vi "Fetch Data (SubVI).vi"(4 "error IN":errorcluster, 7 "query string":string="SELECT * FROM dbo.ThreatCalibers") -> (0 "error OUT":errorcluster, 3 "recordset data":string[][](array[string]))   [LabVIEW 2015]
uses:
  <vilib>/addons/database/Connection.llb/DB Tools Open Connec (Path).vi
  <vilib>/addons/database/Connection.llb/Conn Execute.vi
  <vilib>/addons/database/Recordset.llb/Rec Destroy - Connection.vi
  <vilib>/addons/database/NI_Database_API.lvlib
panel:
  out "App.Dir":path
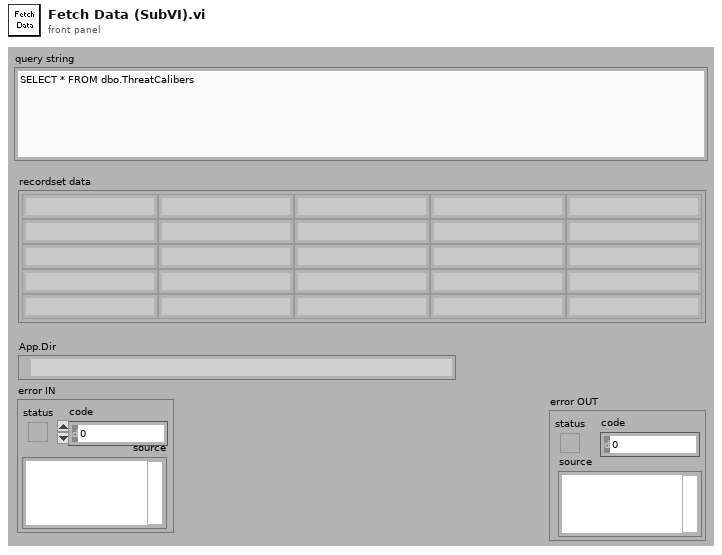
[diagram p1: front panel]
types:
  T1 = typedef "NI_Database_API.lvlib/Conn ObjectReference.ctl" = refnum<k1>
  T2 = typedef "NI_Database_API.lvlib/Rec ObjectReference.ctl" = refnum<k1>
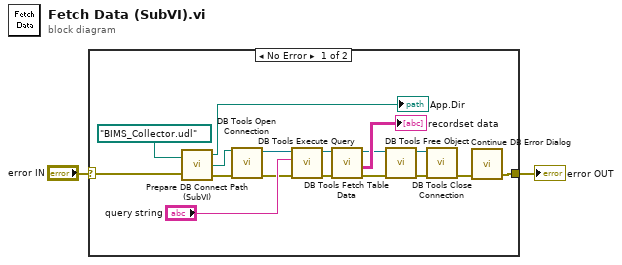
[diagram p0: block diagram]
diagram:
  n1 = case shown="No Error" "error IN" {
    selector: "error IN" -> [w3 w20]
    tunnel: [w19 w20] -> w2
    frame No Error {
      n2 = call "Prepare DB Connect Path (SubVI).vi"("connectString"=path "BIMS_Collector.udl", "error in"=w3) -> ("App.Dir"=→"App.Dir":path, "appended path"=w4:path, "error out"=w6:errorcluster)
      n3 = call-poly <vilib>:"DB Tools Open Connection.vi"("error in (no error)"=w6, "connection information"=w4) -> ("error out"=w12:errorcluster, "connection reference"=w10:T1)  [unwired: 3 in, 3 out]
      n4 = call-poly <vilib>:"DB Tools Execute Query.vi"("error in (no error)"=w12, "SQL query"="query string", "connection reference"=w10) -> ("error out"=w13:errorcluster, "recordset reference"=w9:T2)  [unwired: 1 in, 4 out]
      n5 = call <vilib>:"DB Tools Fetch Table Data.vi"("error in (no error)"=w13, "recordset reference"=w9) -> ("error out"=w14:errorcluster, "recordset data"=→"recordset data":string[][], "recordset reference out"=w8:T2)  [unwired: 3 out]
      n6 = call-poly <vilib>:"DB Tools Free Object.vi"("error in (no error)"=w14, "recordset reference"=w8) -> ("error out"=w15:errorcluster, "connection reference"=w11:T1)  [unwired: 8 out]
      n7 = call <vilib>:"DB Tools Close Connection.vi"("error in (no error)"=w15, "connection reference"=w11) -> ("error out"=w18:errorcluster)  [unwired: 5 out]
      n8 = call "Continue DB Error Dialog.vi"("error in (no error)"=w18) -> ("error out"=w19:errorcluster)  [unwired: 3 in, 2 out]
    }
    frame Error {
    }
  }
  "error OUT" <- w2
